vi "Update objective to matlab server.vi"(8 "error in (no error)":errorcluster, 11 "String":string) -> (0 "error out":errorcluster)   [LabVIEW 2017]
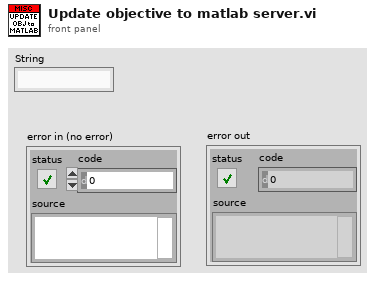
[diagram p1: front panel]
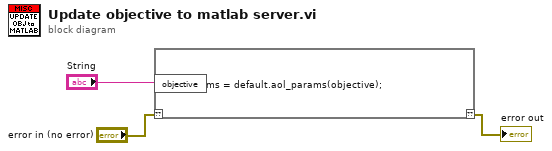
[diagram p0: block diagram]
diagram:
  n1 = script code="aol_params = default.aol_params(objective);"("??"="error in (no error)", "objective"="String") -> ("??"=→"error out":errorcluster)
